vi "ma_Compute t0 eps.vi"   [LabVIEW 2022 SP3, in "NI_MABase.lvlib"]
uses:
  NI_MABase.lvlib
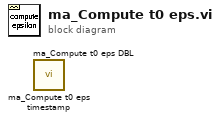
[diagram p0: block diagram]
diagram:
  n1 = call "ma_Compute t0 eps timestamp.vi"() -> ()  [unwired: 11 in, 1 out]
  n2 = call "ma_Compute t0 eps DBL.vi"() -> ()  [unwired: 11 in, 1 out]
